vi "CCD Save Loop.vi"(8 "error in (no error)":cluster{"状态":bool, "代码":i32, "源":string} caption="错误输入（无错误）", 9 "数据通知器":refnum<notifier>, 10 "Save":refnum<queue>, 11 "Director":refnum<queue>) -> (0 "error out":cluster{"状态":bool, "代码":i32, "源":string} caption="错误输出")   [LabVIEW 2015, in "CCD.lvlib"]
doc: "消息循环子VI负责处理与记录数据相关的消息。"
uses:
  CCD.lvlib
  support/Message Queue/Message Cluster.ctl
  <vilib>/vision/Image Controls.llb/IMAQ Image.ctl
  <vilib>/Utility/error.llb/Error Cluster From Error Code.vi
  <vilib>/ErrorRing/Error Ring.xnode
  support/Message Queue/Message Queue.lvlib
  Utility VIs/Utility VIs.lvlib
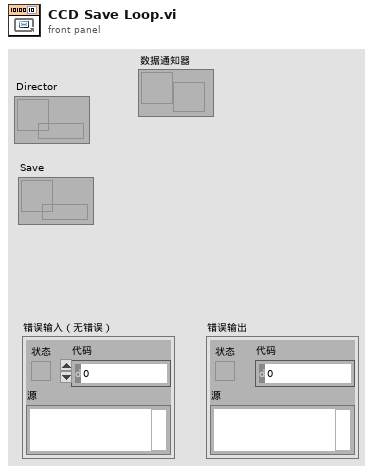
[diagram p1: front panel]
types:
  T1 = typedef "IMAQ Image.ctl" = refnum<image>
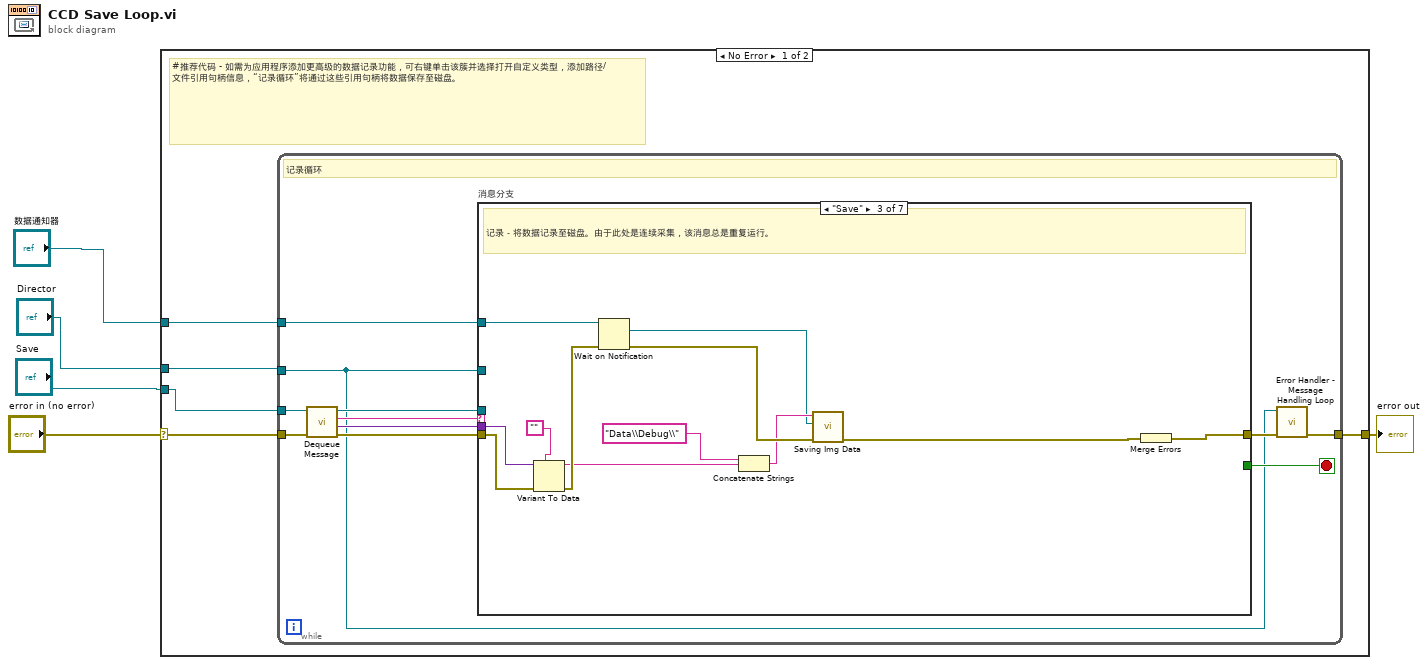
[diagram p0: block diagram]
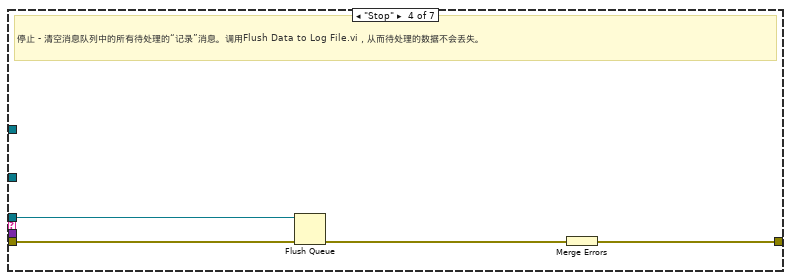
[diagram p4: hidden frame]
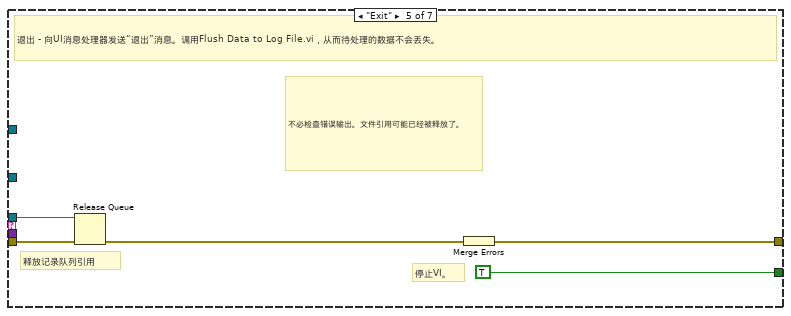
[diagram p5: hidden frame]
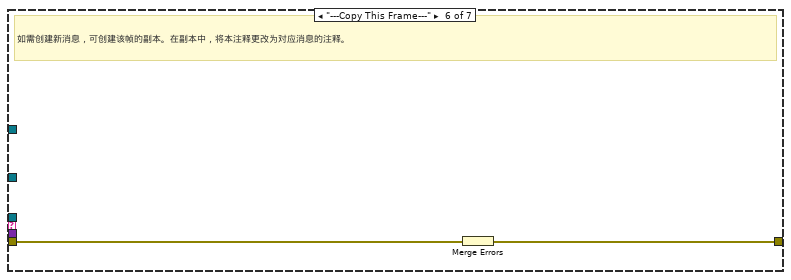
[diagram p6: hidden frame]
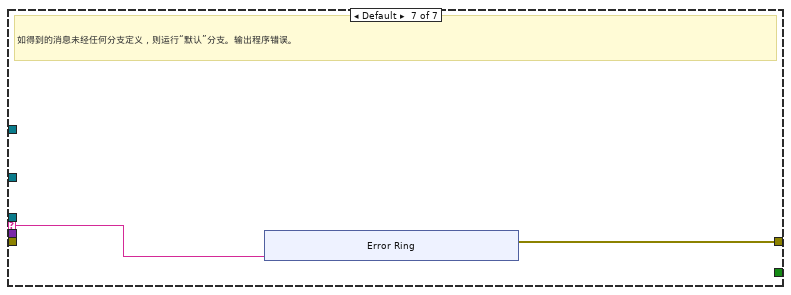
[diagram p7: hidden frame]
diagram:
  n1 = case shown="No Error" "error in (no error)" {
    selector: "error in (no error)" -> [w9 w56]
    tunnel: [w10 w56] -> w5
    tunnel: "数据通知器" -> [w8 _]
    tunnel: "Save" -> [w7 _]
    tunnel: "Director" -> [w6 _]
    frame No Error {
      # "#推荐代码 - 如需为应用程序添加更高级的数据记录功能，可右键单击该簇并选择打开自定义类型，添加路径/文件引用句柄信息，“记录循环”将通过这些引用句柄将数据保存至磁盘。"
      n2 = while {
        tunnel: w7 -> [w15]
        tunnel: w6 -> [w11]
        tunnel: w8 -> [w14]
        tunnel: w9 -> [w20]
        tunnel: [w13] -> w10
        stop <- w21 stop-if-true
        # "记录循环"
        n3 = call "Dequeue Message.vi"("error in (no error)"=w20, "消息队列"=w15) -> ("error out"=w19:cluster{"状态":bool, "代码":i32, "源":string}, "消息数据"=w17:variant, "消息"=w18:string, "消息队列副本"=w16:refnum<queue>)  [unwired: 6 in]
        n4 = case "消息分支" shown="\"Save\"" w18 {
          selector: w18 -> [_ _ _ _ _ _ w47]
          tunnel: w16 -> [_ _ _ w36 w41 _ _]
          tunnel: w19 -> [w22 w23 w32 w37 w42 w46 _]
          tunnel: [w22 w23 w35 w39 w43 w45 w48] -> w12
          tunnel: [_ _ _ _ TRUE _ _] -> w21
          tunnel: w17 -> [_ _ w33 _ _ _ _]
          tunnel: w11 -> [_ _ _ _ _ _ _]
          tunnel: w14 -> [_ _ w34 _ _ _ _]
          frame "Initialize" {
            # "初始化－第一次启动时将被调用。当前不包含任何操作。"
          }
          frame "Start" {
            # "开始 - 发送“记录”消息，开始记录。根据记录文件基路径的值生成一个唯一的带时间标识的TDMS文件名。"
          }
          frame "Save" {
            # "记录－将数据记录至磁盘。由于此处是连续采集，该消息总是重复运行。"
            n5 = Variant To Data(error in=w32, type="", Variant=w33) -> (data=w24:string, error out=w31:errorcluster)
            n6 = Wait on Notification(notifier=w34, error in (no error)=w31) -> (notification=w26:T1, error out=w29:errorcluster)  [unwired: 2 in, 2 out]
            n7 = Concatenate Strings("Data\\Debug\\", w24) -> (w27:string)
            n8 = call "Saving Img Data.vi"("error in (no error)"=w29, "Image"=w26, "名称或相对路径"=w27) -> ("error out"=w28:errorcluster)  [unwired: 8 in]
            n9 = Merge Errors(w28) -> (w35:errorcluster)
          }
          frame "Stop" {
            # "停止 - 清空消息队列中的所有待处理的“记录”消息。调用Flush Data to Log File.vi，从而待处理的数据不会丢失。"
            n10 = Flush Queue(queue=w36, error in (no error)=w37) -> (error out=w38:errorcluster)  [unwired: 2 out]
            n11 = Merge Errors(w38) -> (w39:errorcluster)
          }
          frame "Exit" {
            # "不必检查错误输出。文件引用可能已经被释放了。"
            # "释放记录队列引用"
            # "停止VI。"
            # "退出 - 向UI消息处理器发送“退出”消息。调用Flush Data to Log File.vi，从而待处理的数据不会丢失。"
            n12 = Release Queue(queue=w41, error in (no error)=w42) -> (error out=w40:errorcluster)  [unwired: 1 in, 2 out]
            n13 = Merge Errors(w40) -> (w43:errorcluster)
          }
          frame "---Copy This Frame---" {
            # "如需创建新消息，可创建该帧的副本。在副本中，将本注释更改为对应消息的注释。"
            n14 = Merge Errors(w46) -> (w45:errorcluster)
          }
          frame Default {
            # "如得到的消息未经任何分支定义，则运行“默认”分支。输出程序错误。"
            n15 = xnode ("Error Ring")("parameter 0"=w47) -> ("error out"=w48:errorcluster)
          }
        }
        n16 = call "Error Handler - Message Handling Loop.vi"("error in (no error)"=w12, "消息队列"=w11) -> ("错误输入副本"=w13:cluster{"状态":bool, "代码":i32, "源":string})  [unwired: 8 in, 1 out]
      }
    }
    frame Error {
    }
  }
  "error out" <- w5
